vi "Log_Reference_Velocity.vi"(1 "Measured Velocity":dbl) -> ()   [LabVIEW 2010]
uses:
  Controls/Server_Comms.ctl
  Controls/Post_Process.ctl
  File/Setup_Filetype.ctl
  Globals/Meas_global.vi
  Globals/Preference_global.vi
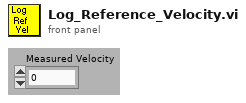
[diagram p1: front panel]
types:
  T1 = typedef "Post_Process.ctl" = enum16{"Take New Data", "Post Process Raw Data File"}
  T2 = typedef "Server_Comms.ctl" = enum16{"Server Link Healthy", "Do Not Link To Server"}
  T3 = typedef "Setup_Filetype.ctl" = enum16{"Measurement Setups", "Calibration Setups", "General", "Results File Plotter Setups", "Speed Calib Tweaks"}
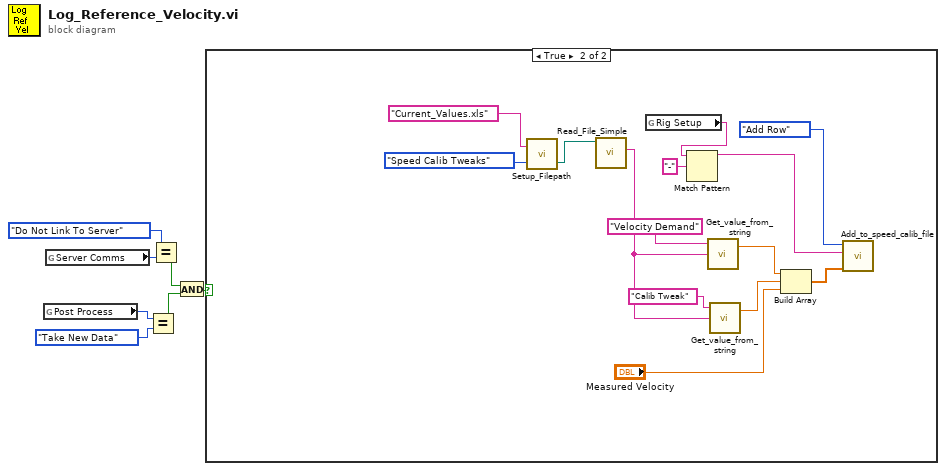
[diagram p0: block diagram]
diagram:
  n1 = global read "Meas_global.vi" "Post Process"() -> (w6:T1)
  n2 = global read "Preference_global.vi" "Server Comms"() -> (w5:T2)
  n3 = Equal?(x=w6, y=Post_Process."Take New Data" ("Post Process")) -> (x = y?=w3:bool)
  n4 = Equal?(x=Server_Comms."Do Not Link To Server" ("Server Comms"), y=w5) -> (x = y?=w2:bool)
  n5 = And(x=w2, y=w3) -> (x .and. y?=w1:bool)
  n6 = case shown="True" w1 {
    frame False {
    }
    frame True {
      n7 = call "Setup_Filepath.vi"("Setup File Type"=Setup_Filetype."Speed Calib Tweaks", "Filename in"="Current_Values.xls" ("name or relative path")) -> ("Filename Out"=w8:path)  [unwired: 1 out]
      n8 = call "Read_File_Simple.vi"("Filename"=w8) -> ("string"=w21:string)  [unwired: 2 in, 7 out]
      n9 = global read "Preference_global.vi" "Rig Setup"() -> (w13:string)
      n10 = Match Pattern(string=w13, regular expression="-") -> (before substring=w11:string)  [unwired: 4 out]
      n11 = call "Get_value_from_string.vi"("Input string"=w21, "Variable name"="Velocity Demand") -> ("Value"=w18:dbl)  [unwired: 1 in, 1 out]
      n12 = call "Get_value_from_string.vi"("Input string"=w21, "Variable name"="Calib Tweak") -> ("Value"=w17:dbl)  [unwired: 1 in, 1 out]
      n13 = Build Array(w18, w17, "Measured Velocity") -> (w15:dbl[])
      n14 = call "Add_to_speed_calib_file.vi"("New Row"=w15, "Rig Name"=w11, "Mode"=enum16{"Add Row", "Get Error Value"}."Add Row") -> ()  [unwired: 3 in, 2 out]
    }
  }
